vi "get_wl.vi"(8 "error in (no error)":errorcluster, 11 "source":enum16{"None", "ch1", "ch2", "ch3", "ch4"}(ring)=enum."ch1") -> (0 "error out":errorcluster, 2 "wl":dbl)   [LabVIEW 2017, in "highfinesse.lvlib"]
uses:
  highfinesse.lvlib
  wlmData.dll
panel:
  out "calls":i32
  in  "retry (ms)":u32=1000
  in  "max_attempts":i32=5
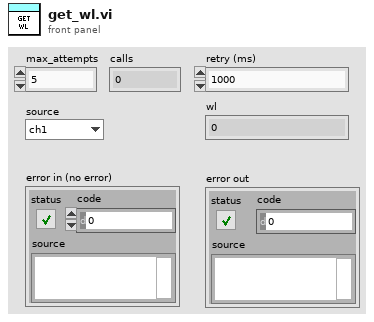
[diagram p1: front panel]
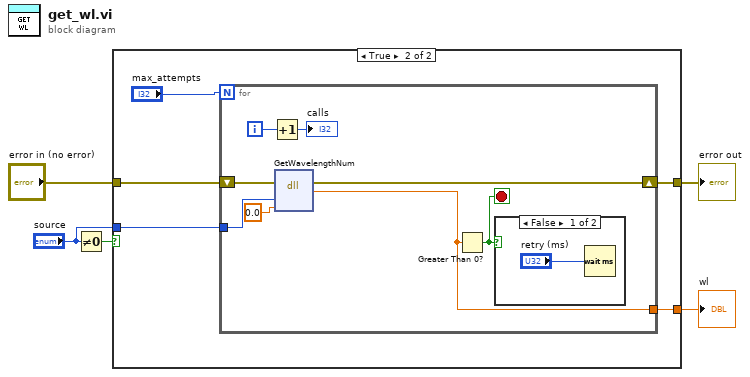
[diagram p0: block diagram]
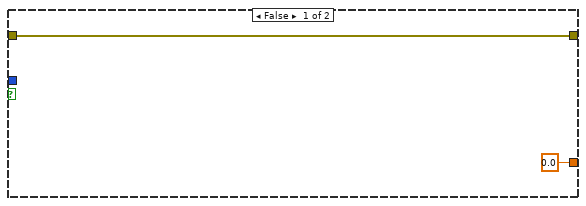
[diagram p2: hidden frame]
diagram:
  n1 = Not Equal To 0?(x="source") -> (x != 0?=w5:bool)
  n2 = case shown="True" w5 {
    tunnel: [w7 w12] -> w3
    tunnel: "error in (no error)" -> [w7 w11]
    tunnel: "source" -> [_ w10]
    tunnel: [0.0 ("return type") w9] -> w2
    frame False {
    }
    frame True {
      n3 = for {
        N: "max_attempts" -> [_]
        tunnel: w10 -> [w17]
        tunnel: [w16] -> w9
        shift-right: [w19] -> w12
        shift-left: w11 -> [w18]
        i -> [w14]
        stop <- w15 stop-if-true
        n4 = Increment(x=w14) -> (x+1=→"calls":i32)
        n5 = dll-call lib="wlmData.dll" fn="GetWavelengthNum"(error in=w18, "arg1"=w17, "arg2"=0.0) -> (error out=w19:errorcluster, "return type"=w16:dbl)  [unwired: 4 in, 1 out]
        n6 = Greater Than 0?(x=w16) -> (x > 0?=w15:bool)
        n7 = case shown="False" w15 {
          frame False {
            n8 = Wait (ms)(milliseconds to wait="retry (ms)") -> ()  [unwired: 1 out]
          }
          frame True {
          }
        }
      }
    }
  }
  "error out" <- w3
  "wl" <- w2
